vi "NewPower_Release.vi"(2 "error in (no error)":errorcluster, 3 "485Port In":refnum<visa-resource-name>="COM3") -> (0 "error out":errorcluster, 1 "485Port Out":refnum<visa-resource-name>)   [LabVIEW 2011]
uses:
  <vilib>/Instr/_visa.llb/VISA Configure Serial Port (Instr).vi
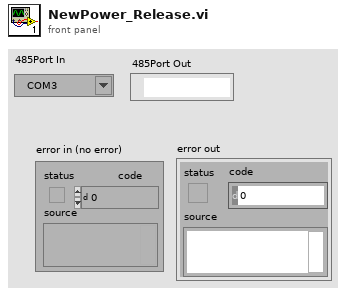
[diagram p1: front panel]
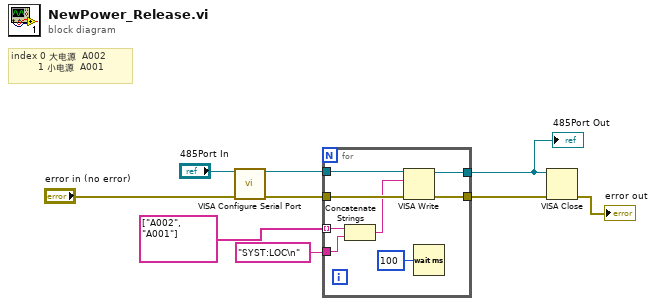
[diagram p0: block diagram]
diagram:
  # "index 0 大电源  A002\n         1 小电源  A001"
  n1 = call-poly "VISA Configure Serial Port"("VISA resource name"="485Port In", "error in (no error)"="error in (no error)") -> ("VISA resource name out"=w8:refnum<visa-resource-name>, "error out"=w7:errorcluster)  [unwired: 12 in]
  n2 = for {
    tunnel: w8 -> [w17]
    tunnel: w7 -> [w16]
    tunnel: string[] ["A002", "A001"] -> [w15] mode=indexing
    tunnel: "SYST:LOC\n" -> [w14]
    tunnel: [w12] -> w1
    tunnel: [w11] -> w4
    n3 = Concatenate Strings(w15, w14) -> (w13:string)
    n4 = VISA Write(VISA resource name=w17, write buffer=w13, error in (no error)=w16) -> (VISA resource name out=w12:refnum<visa-resource-name>, error out=w11:errorcluster)  [unwired: 1 out]
    n5 = Wait (ms)(milliseconds to wait=u32 100) -> ()  [unwired: 1 out]
  }
  "485Port Out" <- w1
  n6 = VISA Close(VISA resource name=w1, error in (no error)=w4) -> (error out=→"error out":errorcluster)
